vi "WZ5005E-Config.vi"(5 "MyIndex":u8, 6 "保护电流(A)":dbl=1.5, 7 "保护电压(V)":dbl=7.0, 8 "error in":errorcluster caption="错误输入（无错误）", 9 "输出电流(A)":dbl=1.0, 10 "输出电压(V)":dbl=5.0, 11 "地址":string="02") -> (0 "error out":errorcluster, 3 "Result":bool)   [LabVIEW 2015, in "WZ5005E.lvlib"]
uses:
  WZ5005E.lvlib
  <vilib>/Instr/_visa.llb/VISA Configure Serial Port (Instr).vi
panel:
  out "VISA":refnum<visa-resource-name>
  out "Send":string
  # "保护设置并不起作用，默认52V，5.2A"
  # "电压只精确到小数点后2位，电流3位"
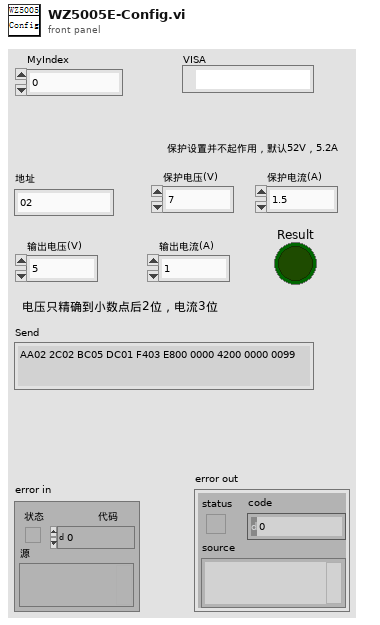
[diagram p1: front panel]
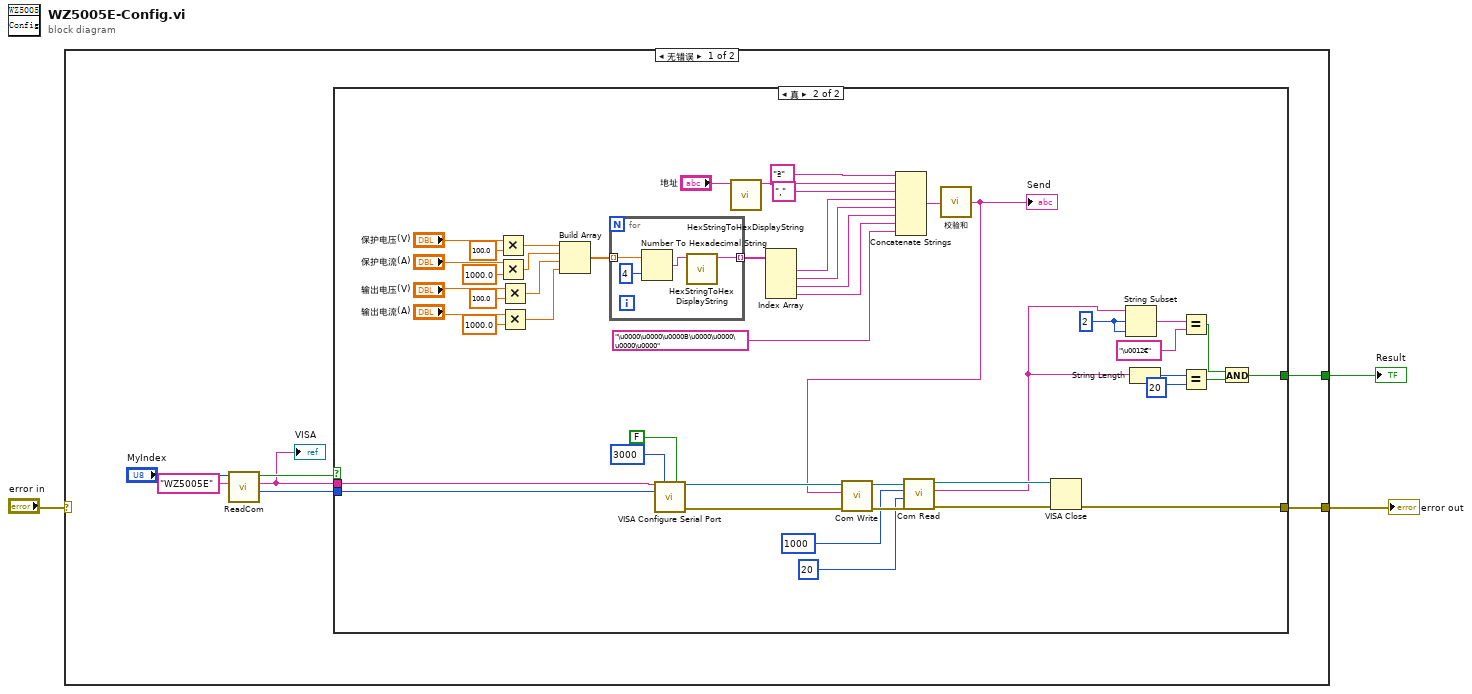
[diagram p0: block diagram]
diagram:
  n1 = case shown="无错误" "error in" {
    selector: "error in" -> [_ w62]
    tunnel: [w10 w62] -> w3
    tunnel: [w4 _] -> w1
    frame No Error {
      n2 = call "ReadCom.vi"("仪器名称"="WZ5005E", "MyIndex"="MyIndex") -> ("Baudrate"=w5:i32, "COM"=w6:string, "OK?"=w7:bool)  [unwired: 7 in]
      "VISA" <- w6
      n3 = case shown="真" w7 {
        tunnel: [_ w57] -> w10
        tunnel: w6 -> [_ w56]
        tunnel: w5 -> [_ w55]
        tunnel: [_ w13] -> w4
        frame False {
        }
        frame True {
          w20 = 2 ("偏移量(0)")
          n4 = Multiply(x="保护电压(V)", y=100.0) -> (x*y=w30:dbl)
          n5 = Multiply(x="保护电流(A)", y=1000.0) -> (x*y=w37:dbl)
          n6 = Multiply(x="输出电压(V)", y=100.0) -> (x*y=w38:dbl)
          n7 = Multiply(x="输出电流(A)", y=1000.0) -> (x*y=w39:dbl)
          n8 = Build Array(w30, w37, w38, w39) -> (w40:dbl[])
          n9 = for {
            tunnel: w40 -> [w59] mode=indexing
            tunnel: [w60] -> w41 mode=indexing
            n10 = Number To Hexadecimal String(1:i16 4 ("宽度(-)"), 2:w59) -> (0:w61:string)
            n11 = call "HexStringToHexDisplayString.vi"("正常显示HEX字符串"=w61) -> ("HEX显示字符串"=w60:string)  [unwired: 10 in]
          }
          n12 = call-poly "VISA Configure Serial Port"("VISA resource name"=w56, "timeout (10sec)"=u32 3000, "Enable Termination\nChar (T)"=FALSE ("Enable Termination\nChar (T)"), "baud rate (9600)"=w55) -> ("VISA resource name out"=w53:refnum<visa-resource-name>, "error out"=w52:errorcluster)  [unwired: 10 in]
          n13 = call "HexStringToHexDisplayString.vi"("正常显示HEX字符串"="地址") -> ("HEX显示字符串"=w25:string)  [unwired: 10 in]
          n14 = Index Array(array=w41) -> (element #1=w42:string, element #2=w43:string, element #3=w44:string, element #4=w45:string)  [unwired: 4 in]
          n15 = Concatenate Strings("ª", w25, ",", w42, w43, w44, w45, "\u0000\u0000\u0000B\u0000\u0000\u0000\u0000") -> (w27:string)
          n16 = call "校验和.vi"("输入（Hex）"=w27) -> ("输出"=w22:string)
          "Send" <- w22
          n17 = call "Com Write.vi"("错误输入（无错误）"=w52, "Wbuff"=w22, "VISA In"=w53) -> ("错误输出"=w50:errorcluster, "VISA Out"=w51:refnum<visa-resource-name>)  [unwired: 6 in, 1 out]
          n18 = call "Com Read.vi"("错误输入（无错误）"=w50, "num"=u32 20, "超时"=u32 1000, "VISA In"=w51) -> ("错误输出"=w49:errorcluster, "buff"=w14:string, "VISA Out"=w48:refnum<visa-resource-name>)  [unwired: 4 in, 1 out]
          n19 = VISA Close(VISA resource name=w48, error in (no error)=w49) -> (error out=w57:errorcluster)
          n20 = String Subset(string=w14, offset (0)=w20, length (rest)=w20) -> (substring=w19:string)
          n21 = String Length(string=w14) -> (length=w15:i32)
          n22 = Equal?(x=w19, y="\u0012€" ("正则表达式")) -> (x = y?=w21:bool)
          n23 = Equal?(x=w15, y=20) -> (x = y?=w17:bool)
          n24 = And(x=w21, y=w17) -> (x .and. y?=w13:bool)
        }
      }
    }
    frame Error {
    }
  }
  "error out" <- w3
  "Result" <- w1
